vi "Initialize.vi"(5 "components directory":path, 7 "options":T1, 8 "error in (no error)":errorcluster, 10 "framework configuration":T6, 11 "VeriStand Data Sharing Framework in":refnum<class "VeriStand Data Sharing Framework.lvclass">=refnum) -> (0 "error out":errorcluster, 3 "VeriStand Data Sharing Framework out":refnum<class "VeriStand Data Sharing Framework.lvclass">)   [LabVIEW 2017, in "Data Sharing Framework Engine.lvlib" / "VeriStand Data Sharing Framework.lvclass"]
uses:
  VeriStand Data Sharing Framework.lvclass
  DSF Core.lvlibp/DSF Configuration API/Public/Controls/DSF Engine Framework Configuration.ctl
  DSF Core.lvlibp/DSF Configuration API/Public/Controls/DSF Engine Plugin Configuration.ctl
  DSF Core.lvlibp/DSF Configuration API/Public/Controls/DSF Timing Info.ctl
  DSF Core.lvlibp/DSF Configuration API/Public/Controls/DSF Engine Plugin Thread Configuration.ctl
  DSF Core.lvlibp/DSF Configuration API/Public/Controls/DSF Settings Info.ctl
  DSF Core.lvlibp/DSF Configuration API/Public/Controls/DSF Engine Transfer Group Configuration.ctl
  DSF Core.lvlibp/DSF Configuration API/Public/Controls/DSF Direction.ctl
  DSF Core.lvlibp/DSF Configuration API/Public/Controls/DSF Engine Transfer Configuration.ctl
  DSF Core.lvlibp/DSF Configuration API/Public/Controls/DSF Byte Order.ctl
  DSF Core.lvlibp/DSF Configuration API/Public/Controls/DSF Engine Channel Configuration.ctl
  DSF Core.lvlibp/DSF Configuration API/Public/Controls/DSF Data Type.ctl
  DSF Core.lvlibp/DSF Configuration API/Public/Controls/DSF Timeout Behavior.ctl
  DSF Core.lvlibp/Engine/Classes/Framework/Framework Options.ctl
  DSF Core.lvlibp/Engine/Typedefs/FIFO Flags.ctl
  DSF Core.lvlibp/Engine/Classes/Thread/Thread Options.ctl
  DSF Core.lvlibp/Engine/Typedefs/Plugin Flags.ctl
  DSF Core.lvlibp/Engine/Typedefs/Performance Options.ctl
  DSF Core.lvlibp/Engine/Classes/Framework/Framework.lvclass
  C:/Git/DSF/VeriStand Data Sharing Custom Device/Data Sharing Custom Device/Source/Engine/DSF Core.lvlibp/Engine/Classes/Framework/Framework.lvclass
  DSF Core.lvlibp
  DSF Core.lvlibp/Engine/Classes/Status/Performance.lvclass
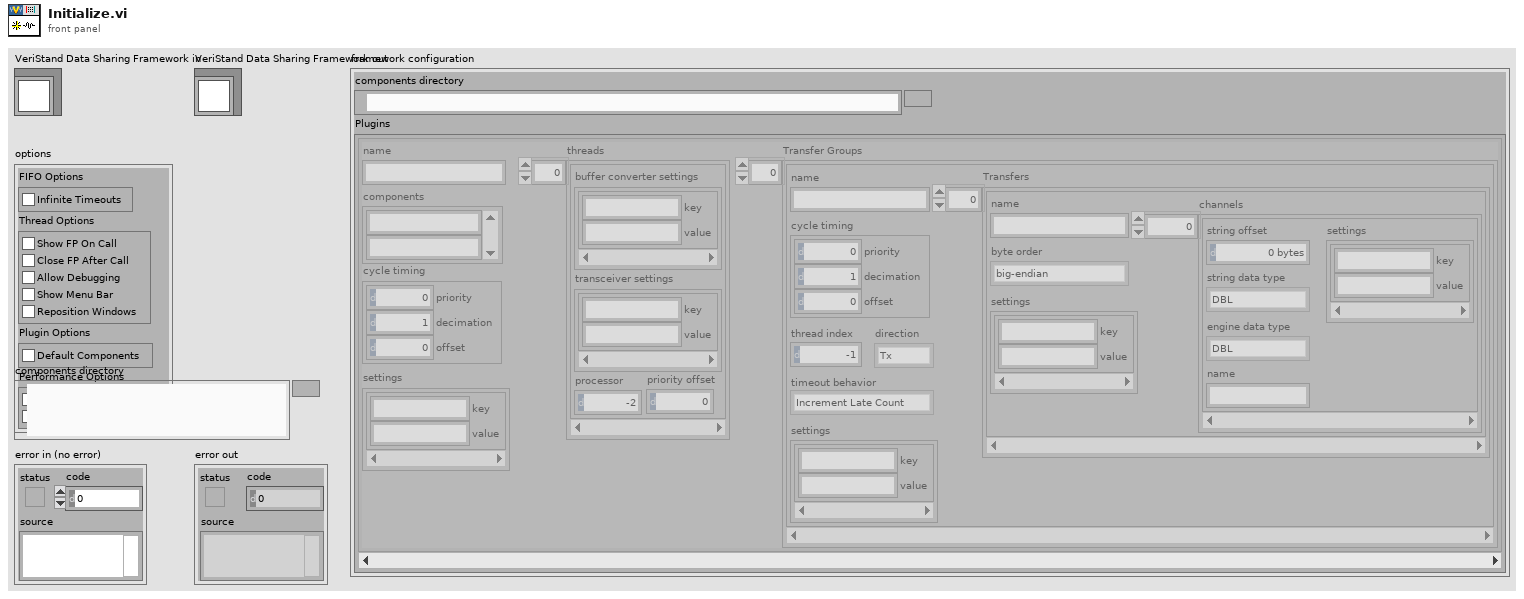
[diagram p1: front panel]
types:
  T1 = typedef "DSF Core.lvlibp/Framework.lvclass/Framework Options.ctl" = cluster{"FIFO Options":T2, "Thread Options":T3, "Plugin Options":T4, "Performance Options":T5}
  T2 = typedef "DSF Core.lvlibp/FIFO Flags.ctl" = cluster{"Infinite Timeouts":bool}
  T3 = typedef "DSF Core.lvlibp/Thread Options.ctl" = cluster{"Show FP On Call":bool, "Close FP After Call":bool, "Allow Debugging":bool, "Show Menu Bar":bool, "Reposition Windows":bool}
  T4 = typedef "DSF Core.lvlibp/Plugin Flags.ctl" = cluster{"Default Components":bool}
  T5 = typedef "DSF Core.lvlibp/Performance.lvclass/Performance Options.ctl" = cluster{"Measure Period":bool, "Measure Rx/Tx Duration":bool}
  T6 = typedef "DSF Core.lvlibp/DSF Engine Framework Configuration.ctl" = cluster{"components directory":path, "Plugins":T7[]}
  T7 = typedef "DSF Core.lvlibp/DSF Engine Plugin Configuration.ctl" = cluster{"name":string, "components":string[], "cycle timing":T8, "threads":T9[], "Transfer Groups":T11[], "settings":T10}
  T8 = typedef "DSF Core.lvlibp/DSF Timing Info.ctl" = cluster{"priority":u64, "decimation":u64, "offset":u64}
  T9 = typedef "DSF Core.lvlibp/DSF Engine Plugin Thread Configuration.ctl" = cluster{"buffer converter settings":T10, "transceiver settings":T10, "processor":i32, "priority offset":i16}
  T10 = typedef "DSF Core.lvlibp/DSF Settings Info.ctl" = cluster{"key":string, "value":string}[]
  T11 = typedef "DSF Core.lvlibp/DSF Engine Transfer Group Configuration.ctl" = cluster{"name":string, "direction":T12, "cycle timing":T8, "thread index":i32, "settings":T10, "Transfers":T13[], "timeout behavior":T17}
  T12 = typedef "DSF Core.lvlibp/DSF Direction.ctl" = enum8{"Tx", "Rx"}
  T13 = typedef "DSF Core.lvlibp/DSF Engine Transfer Configuration.ctl" = cluster{"name":string, "byte order":T14, "settings":T10, "channels":T15[]}
  T14 = typedef "DSF Core.lvlibp/DSF Byte Order.ctl" = enum8{"big-endian", "little-endian"}
  T15 = typedef "DSF Core.lvlibp/DSF Engine Channel Configuration.ctl" = cluster{"string offset":u64, "string data type":T16, "engine data type":T16, "name":string, "settings":T10}
  T16 = typedef "DSF Core.lvlibp/DSF Data Type.ctl" = enum8{"Bool", "SGL", "DBL", "I8", "I16", "I32", "I64", "U8", "U16", "U32", "U64"}
  T17 = typedef "DSF Core.lvlibp/DSF Timeout Behavior.ctl" = enum8{"Increment Late Count", "Throw Error"}
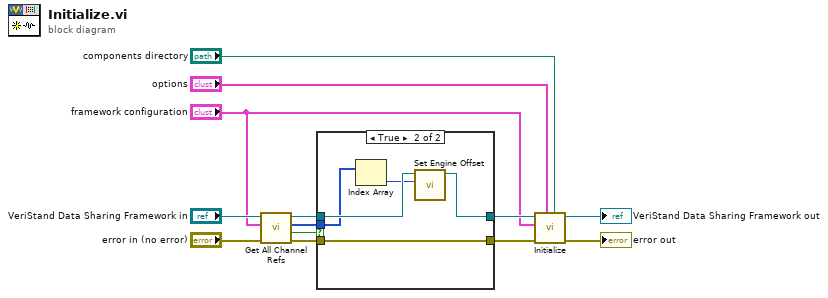
[diagram p0: block diagram]
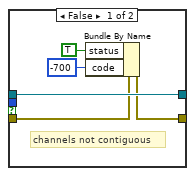
[diagram p2: hidden frame]
diagram:
  n1 = call "Get All Channel Refs.vi"("error in (no error)"="error in (no error)", "framework configuration in"="framework configuration", "VeriStand Data Sharing Framework in"="VeriStand Data Sharing Framework in") -> ("error out"=w10:errorcluster, "contiguous?"=w6:bool, "all channel offsets"=w7:u64[], "VeriStand Data Sharing Framework out"=w8:refnum<class "VeriStand Data Sharing Framework.lvclass">)  [unwired: 5 in]
  n2 = case shown="True" w6 {
    tunnel: [w14 w23] -> w2
    tunnel: [w18 w19] -> w3
    tunnel: w10 -> [w17 w23]
    tunnel: w8 -> [w18 w22]
    tunnel: w7 -> [_ w20]
    frame False {
      # "channels not contiguous"
      n3 = Bundle By Name(cluster=w17, "status"=TRUE, "code"=-700) -> (w14:errorcluster)
    }
    frame True {
      n4 = Index Array(array=w20) -> (element=w21:u64)  [unwired: 1 in]
      n5 = call "Set Engine Offset.vi"("engine offset"=w21, "Framework in"=w22) -> ("Framework out"=w19:refnum<class "VeriStand Data Sharing Framework.lvclass">)  [unwired: 9 in]
    }
  }
  n6 = call-parent "Initialize.vi"("components directory"="components directory", "options"="options", "error in (no error)"=w2, "framework configuration"="framework configuration", "Framework in"=w3) -> ("error out"=→"error out":errorcluster, "Framework out"=→"VeriStand Data Sharing Framework out":refnum<class "VeriStand Data Sharing Framework.lvclass">)  [unwired: 5 in]
